vi "getAsDictionary.vi"(8 "error in (no error)":errorcluster, 11 "IEnumerationType in":refnum<class "IEnumerationType.lvclass">) -> (0 "error out":errorcluster, 2 "Dictionary out":map{string, i32}(c390), 3 "IEnumerationType out":refnum<class "IEnumerationType.lvclass">)   [LabVIEW 2022 SP3, in "openDAQ.lvlib" / "daqCoreTypes.lvlib" / "IEnumerationType.lvclass"]
uses:
  <instrlib>/openDAQ/Public/Classes/daqCoreTypes/IEnumerationType/IEnumerationType.lvclass
  <instrlib>/openDAQ/Public/Classes/daqCoreTypes/IEnumerationType/IEnumerationType.lvclass/IEnumerationType.ctl
  <instrlib>/openDAQ/Public/Classes/daqCoreTypes/IDict/IDict.lvclass
  <instrlib>/openDAQ/Binaries/Windows/x86/copendaq32.dll
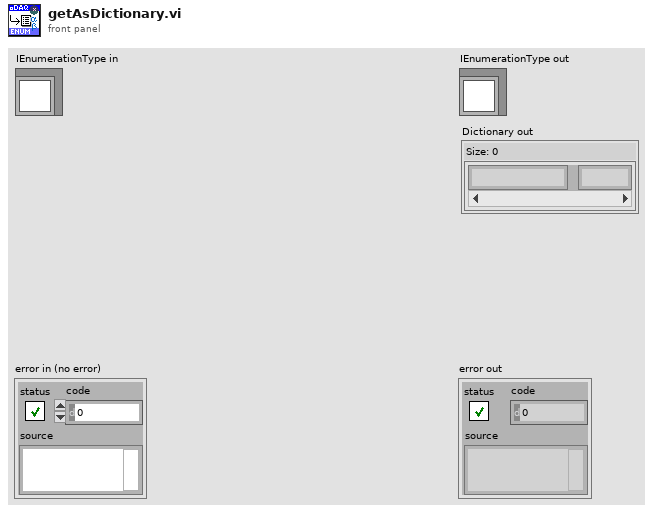
[diagram p1: front panel]
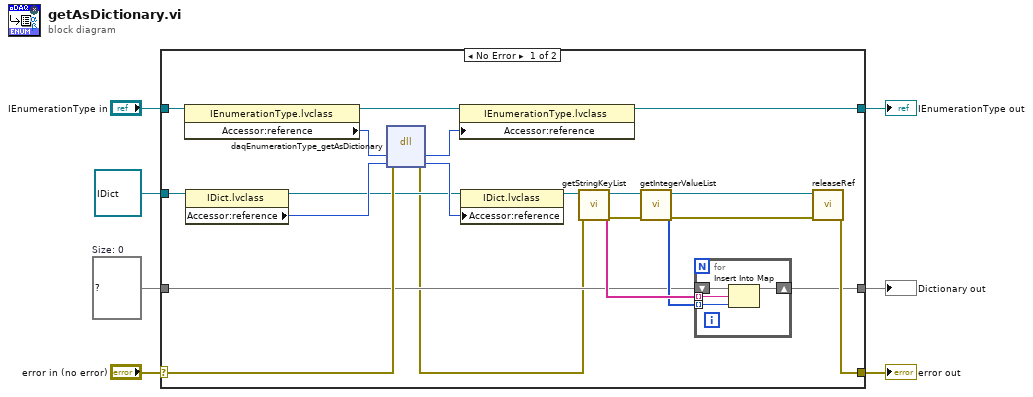
[diagram p0: block diagram]
diagram:
  w2 = map{string, i32} {}  # Size: 0
  n1 = case shown="No Error" "error in (no error)" {
    selector: "error in (no error)" -> [w26 w35]
    tunnel: [w9 w35] -> w6
    tunnel: [w22 w34] -> w4
    tunnel: "IEnumerationType in" -> [w27 w34]
    tunnel: refnum<class "IDict.lvclass"> refnum ("openDAQ.lvlib:daqCoreTypes.lvlib:IDict.lvclass") -> [w21 w33]
    tunnel: [w8 w33] -> w1
    tunnel: w2 -> [w13 _]
    frame No Error {
      n2 = property class="IEnumerationType.lvclass"(reference=w27) -> (reference out=w23:refnum<class "IEnumerationType.lvclass">, "Accessor:reference"=w25:i64)  [unwired: 1 in, 1 out]
      n3 = property class="IDict.lvclass"(reference=w21) -> (reference out=w19:refnum<class "IDict.lvclass">, "Accessor:reference"=w20:i64)  [unwired: 1 in, 1 out]
      n4 = dll-call lib="C:/Program Files (x86)/National Instruments/LabVIEW 2022/instr.lib/openDAQ/Binaries/Windows/x86/copendaq*.*" fn="daqEnumerationType_getAsDictionary"(error in=w26, "enumerationType"=w25, "dictionary"=w20) -> (error out=w11:errorcluster, "enumerationType"=w24:i64, "dictionary"=w28:i64)  [unwired: 3 in, 1 out]
      n5 = property class="IEnumerationType.lvclass"(reference=w23, "Accessor:reference"=w24) -> (reference out=w22:refnum<class "IEnumerationType.lvclass">)  [unwired: 1 in, 1 out]
      n6 = property class="IDict.lvclass"(reference=w19, "Accessor:reference"=w28) -> (reference out=w18:refnum<class "IDict.lvclass">)  [unwired: 1 in, 1 out]
      n7 = call <instrlib>:"getStringKeyList.vi"("error in (no error)"=w11, "IDict in"=w18) -> ("error out"=w16:errorcluster, "Key List out"=w15:string[], "IDict out"=w17:refnum<class "IDict.lvclass">)  [unwired: 7 in]
      n8 = call <instrlib>:"getIntegerValueList.vi"("error in (no error)"=w16, "IDict in"=w17) -> ("error out"=w10:errorcluster, "Integer Value list out"=w14:i32[], "IDict out"=w12:refnum<class "IDict.lvclass">)  [unwired: 7 in]
      n9 = for {
        shift-right: [w31] -> w8
        shift-left: w13 -> [w32]
        tunnel: w15 -> [w30] mode=indexing
        tunnel: w14 -> [w29] mode=indexing
        n10 = Insert Into Map(map in=w32, key=w30, value=w29) -> (map out=w31:map{string, i32})  [unwired: 2 out]
      }
      n11 = call-dynamic "releaseRef.vi"("error in (no error)"=w10, "IBaseObject in"=w12) -> ("error out"=w9:errorcluster)  [unwired: 9 in]
    }
    frame Error {
    }
  }
  "error out" <- w6
  "IEnumerationType out" <- w4
  "Dictionary out" <- w1
